vi "front_microStep.vi"(0 "Zeta_l":i32, 1 "Step":i32, 2 "Stop Mode":string(combo), 3 "Delay":i32, 5 "Zeta_R":i32, 7 "L_Taget_Zeta":i32, 9 "R_Taget_Zeta":i32, 10 "Sensor":enum16{"l", "r", "both"}(ring), 11 "IR_R":dbl, 12 "taget_IR_R":dbl, 13 "IR_L":dbl, 14 "taget_IR_L":dbl, 15 "precision":dbl) -> (4 "OZeta_l":i32, 6 "Ozeta_r":i32, 8 "Done":bool)   [LabVIEW 2017]
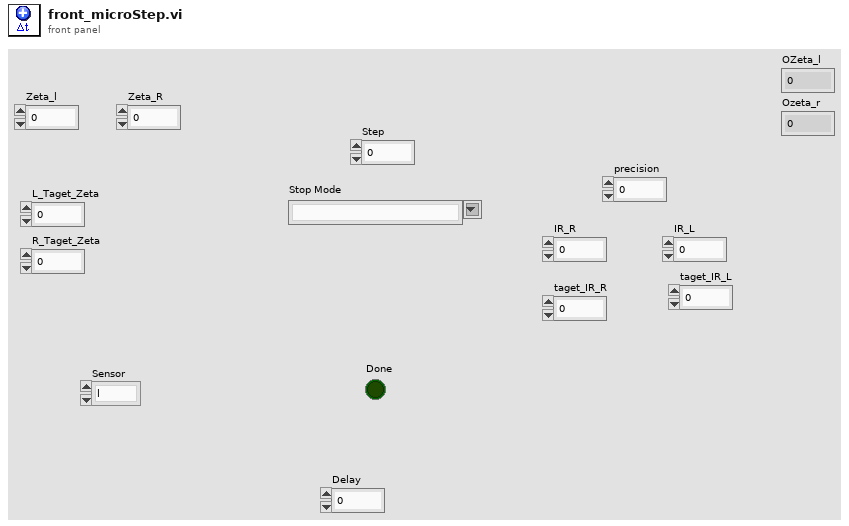
[diagram p1: front panel]
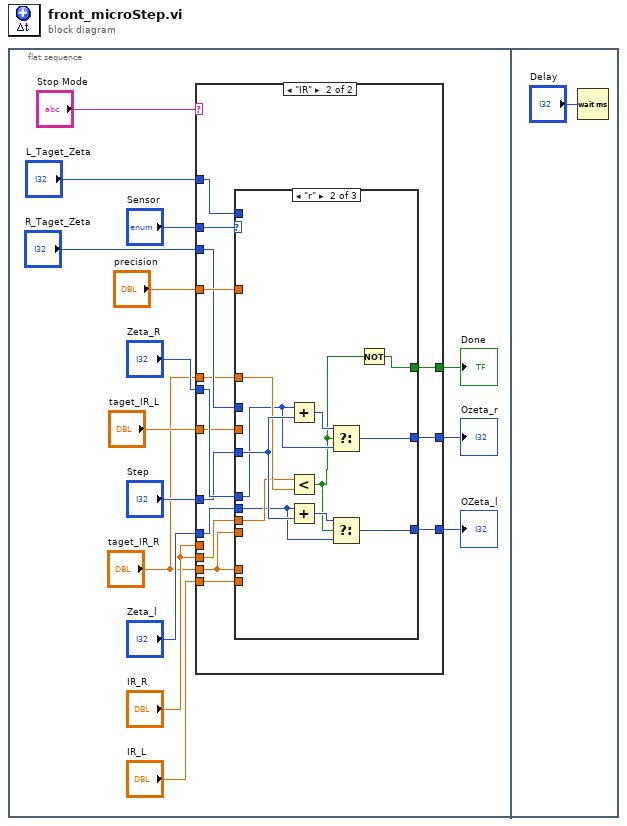
[diagram p0: block diagram]
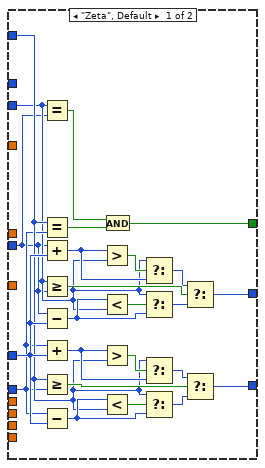
[diagram p2: hidden frame]
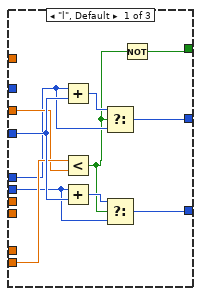
[diagram p3: hidden frame]
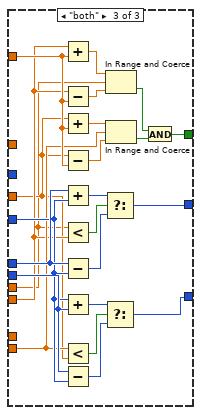
[diagram p4: hidden frame]
diagram:
  n1 = flat-sequence {
    frame #0 {
      n2 = case shown="\"IR\"" "Stop Mode" {
        tunnel: "Zeta_l" -> [w21 w51]
        tunnel: "L_Taget_Zeta" -> [w22 w44]
        tunnel: "Step" -> [w29 w50]
        tunnel: [w27 w53] -> w11
        tunnel: "Zeta_R" -> [w19 w52]
        tunnel: "R_Taget_Zeta" -> [w20 w43]
        tunnel: [w24 w54] -> w8
        tunnel: "IR_R" -> [_ _]
        tunnel: [w18 w49] -> w7
        tunnel: "IR_L" -> [_ w47]
        tunnel: "precision" -> [_ w48]
        tunnel: "taget_IR_R" -> [_ w42]
        tunnel: "taget_IR_L" -> [_ w46]
        tunnel: "Sensor" -> [_ w45]
        tunnel: "IR_R" -> [_ w41]
        tunnel: "taget_IR_R" -> [_ w40]
        frame "Zeta", Default {
          n3 = Equal?(x=w20, y=w19) -> (x = y?=w17:bool)
          n4 = Equal?(x=w22, y=w21) -> (x = y?=w16:bool)
          n5 = Add(x=w19, y=w29) -> (x+y=w38:i32)
          n6 = Greater Or Equal?(x=w20, y=w19) -> (x >= y?=w28:bool)
          n7 = Subtract(x=w19, y=w29) -> (x-y=w34:i32)
          n8 = Add(x=w21, y=w29) -> (x+y=w39:i32)
          n9 = Greater Or Equal?(x=w22, y=w21) -> (x >= y?=w32:bool)
          n10 = Subtract(x=w21, y=w29) -> (x-y=w23:i32)
          n11 = Greater?(x=w38, y=w20) -> (0:w36:bool)
          n12 = Less?(x=w34, y=w20) -> (x < y?=w35:bool)
          n13 = Greater?(x=w39, y=w22) -> (0:w37:bool)
          n14 = Less?(x=w23, y=w22) -> (x < y?=w33:bool)
          n15 = And(x=w17, y=w16) -> (x .and. y?=w18:bool)
          n16 = Select(t=w20, s=w36, f=w38) -> (s? t:f=w26:i32)
          n17 = Select(t=w20, s=w35, f=w34) -> (s? t:f=w25:i32)
          n18 = Select(t=w22, s=w37, f=w39) -> (s? t:f=w31:i32)
          n19 = Select(t=w22, s=w33, f=w23) -> (s? t:f=w30:i32)
          n20 = Select(t=w26, s=w28, f=w25) -> (s? t:f=w24:i32)
          n21 = Select(t=w31, s=w32, f=w30) -> (s? t:f=w27:i32)
        }
        frame "IR" {
          n22 = case shown="\"r\"" w45 {
            tunnel: [w62 w74 w98] -> w54
            tunnel: [w61 w73 w96] -> w53
            tunnel: w52 -> [w57 w68 w93]
            tunnel: w51 -> [w58 w69 w90]
            tunnel: w50 -> [w63 w72 w89]
            tunnel: [w56 w67 w88] -> w49
            tunnel: w48 -> [_ _ w81]
            tunnel: w47 -> [w60 _ w80]
            tunnel: w42 -> [_ _ w79]
            tunnel: w46 -> [w59 _ w78]
            tunnel: w44 -> [_ _ _]
            tunnel: w43 -> [_ _ _]
            tunnel: w42 -> [_ _ _]
            tunnel: w41 -> [_ w70 w77]
            tunnel: w40 -> [_ w71 _]
            frame "l", Default {
              n23 = Add(x=w57, y=w63) -> (x+y=w65:i32)
              n24 = Less?(x=w60, y=w59) -> (x < y?=w55:bool)
              n25 = Add(x=w58, y=w63) -> (x+y=w64:i32)
              n26 = Select(t=w65, s=w55, f=w57) -> (s? t:f=w62:i32)
              n27 = Select(t=w64, s=w55, f=w58) -> (s? t:f=w61:i32)
              n28 = Not(x=w55) -> (.not. x?=w56:bool)
            }
            frame "r" {
              n29 = Add(x=w68, y=w72) -> (x+y=w76:i32)
              n30 = Less?(x=w70, y=w71) -> (x < y?=w66:bool)
              n31 = Add(x=w69, y=w72) -> (x+y=w75:i32)
              n32 = Select(t=w76, s=w66, f=w68) -> (s? t:f=w74:i32)
              n33 = Select(t=w75, s=w66, f=w69) -> (s? t:f=w73:i32)
              n34 = Not(x=w66) -> (.not. x?=w67:bool)
            }
            frame "both" {
              n35 = Add(x=w79, y=w81) -> (x+y=w83:dbl)
              n36 = Subtract(x=w79, y=w81) -> (x-y=w82:dbl)
              n37 = Add(x=w78, y=w81) -> (x+y=w85:dbl)
              n38 = Subtract(x=w78, y=w81) -> (x-y=w84:dbl)
              n39 = Add(x=w93, y=w89) -> (x+y=w99:i32)
              n40 = Less?(x=w77, y=w79) -> (x < y?=w95:bool)
              n41 = Subtract(x=w93, y=w89) -> (x-y=w92:i32)
              n42 = Add(x=w89, y=w90) -> (x+y=w97:i32)
              n43 = Less?(x=w80, y=w78) -> (x < y?=w94:bool)
              n44 = Subtract(x=w90, y=w89) -> (x-y=w91:i32)
              n45 = Select(t=w99, s=w95, f=w92) -> (s? t:f=w98:i32)
              n46 = Select(t=w97, s=w94, f=w91) -> (s? t:f=w96:i32)
              n47 = In Range and Coerce(upper limit=w83, x=w77, lower limit=w82) -> (In Range?=w86:bool)  [unwired: 1 out]
              n48 = In Range and Coerce(upper limit=w85, x=w80, lower limit=w84) -> (In Range?=w87:bool)  [unwired: 1 out]
              n49 = And(x=w86, y=w87) -> (x .and. y?=w88:bool)
            }
          }
        }
      }
      "OZeta_l" <- w11
      "Ozeta_r" <- w8
      "Done" <- w7
    }
    frame #1 {
      n50 = Wait (ms)(milliseconds to wait="Delay") -> ()  [unwired: 1 out]
    }
  }
